vi "Set Swerve Offsets.vi"(0 "Reset Swerve":bool) -> ()   [LabVIEW 2016]
uses:
  <vilib>/Rock Robotics/Network Tables/NT Read Boolean.vi
panel:
  out "Done":bool
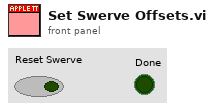
[diagram p1: front panel]
types:
  T1 = typedef "WPI_MotorControlDeviceRef.ctl" = cluster{"DeviceStatus":errorcluster, "Type":T2, "PWM":cluster{"PWM Channel":T3, "DeadBand":T4}, "CAN":cluster{"Device Number":u8, "SetOutput VI Ref":variant, "GetOutput VI Ref":variant, "Enable VI Ref":variant, "Disable VI Ref":variant, "Data":variant}, "Invert":bool}
  T2 = typedef "WPI_MotorControlType.ctl" = enum16{"PWM", "CAN"}
  T3 = typedef "FPGA_DIOPWMChannel.ctl" = enum8{"PWM 0", "PWM 1", "PWM 2", "PWM 3", "PWM 4", "PWM 5", "PWM 6", "PWM 7", "PWM 8", "PWM 9", "PWM MXP 0", "PWM MXP 1", "PWM MXP 2", "PWM MXP 3", "PWM MXP 4", "PWM MXP 5", "PWM MXP 6", "PWM MXP 7", "PWM MXP 8", "PWM MXP 9", "Invalid"}
  T4 = typedef "WPI_PWMDeadband.ctl" = cluster{"Name":string, "maxPositivePwm":i32, "minPositivePwm":i32, "centerPwm":i32, "maxNegativePwm":i32, "minNegativePwm":i32, "angularRange":u16}
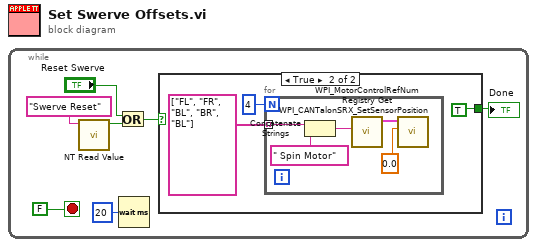
[diagram p0: block diagram]
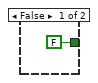
[diagram p2: hidden frame]
diagram:
  n1 = while {
    stop <- FALSE stop-if-true
    n2 = call-poly <vilib>:"NT Read Value.vi"("Name"="Swerve Reset") -> ("Boolean"=w2:bool)  [unwired: 9 in, 1 out]
    n3 = Or(x="Reset Swerve", y=w2) -> (x .or. y?=w4:bool)
    n4 = Wait (ms)(milliseconds to wait=u32 20) -> ()  [unwired: 1 out]
    n5 = case shown="True" w4 {
      tunnel: [FALSE TRUE] -> w5
      frame False {
      }
      frame True {
        n6 = for {
          N: 4 -> [_]
          tunnel: string[] ["FL", "FR", "BL", "BR", "BL"] -> [w15] mode=indexing
          n7 = Concatenate Strings(w15, " Spin Motor" ("string")) -> (w16:string)
          n8 = call <vilib>:"WPI_MotorControlRefNum Registry Get.vi"("refnum name"=w16) -> ("MotorControlDevRef"=w13:T1)  [unwired: 9 in, 1 out]
          n9 = call <vilib>:"WPI_CANTalonSRX_SetSensorPosition.vi"("New Sensor Position"=0.0, "CAN Talon SRX Ref"=w13) -> ()  [unwired: 8 in, 2 out]
        }
      }
    }
    "Done" <- w5
  }
